vi "RegloAnalog.vi"(9 "REGLO D":dbl, 10 "REGLO D 2":dbl, 11 "REGLO D 3":dbl) -> ()   [LabVIEW 2017]
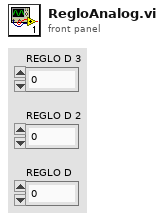
[diagram p1: front panel]
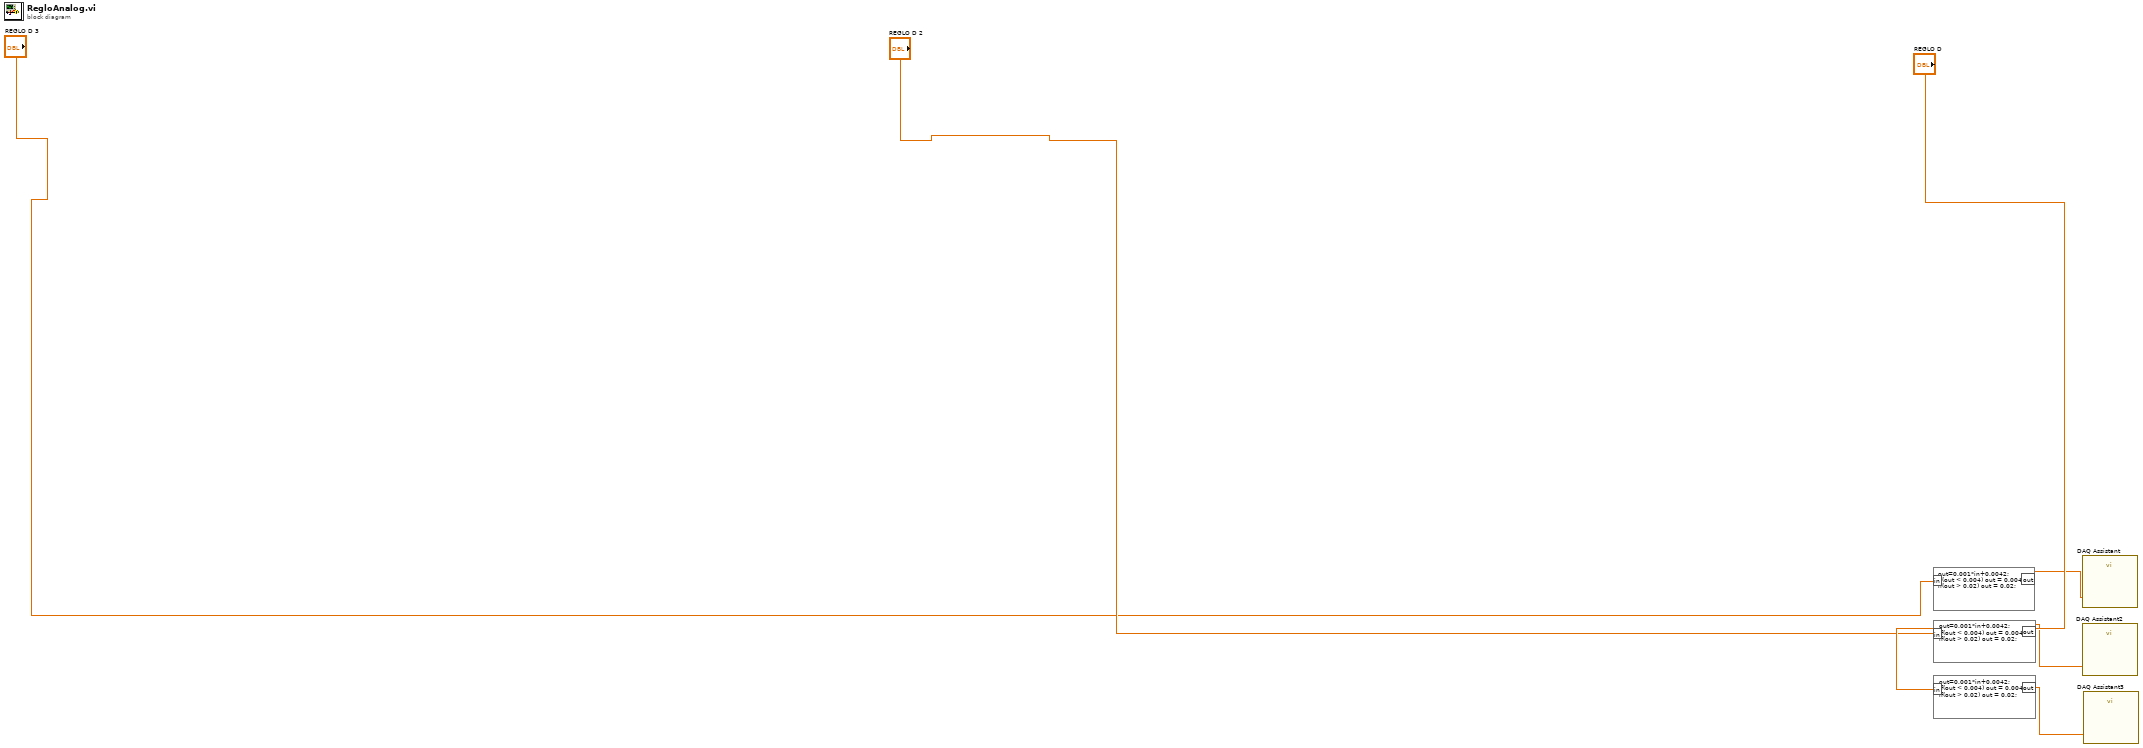
[diagram p0: block diagram]
diagram:
  n1 = formula code="out=0.001*in+0.0042;\nif(out < 0.004) out = 0.0042;\nif(out > 0.02) out = 0.02;"("in"="REGLO D 3") -> ("out"=w2:dbl)
  n2 = formula code="out=0.001*in+0.0042;\nif(out < 0.004) out = 0.0042;\nif(out > 0.02) out = 0.02;"("in"="REGLO D 2") -> ("out"=w4:dbl)
  n3 = formula code="out=0.001*in+0.0042;\nif(out < 0.004) out = 0.0042;\nif(out > 0.02) out = 0.02;"("in"="REGLO D") -> ("out"=w6:dbl)
  n4 = call "DAQ Assistant"("data"=w2) -> ()  [unwired: 17 in, 2 out]
  n5 = call "DAQ Assistant2"("data"=w4) -> ()  [unwired: 17 in, 2 out]
  n6 = call "DAQ Assistant3"("data"=w6) -> ()  [unwired: 17 in, 2 out]
